vi "Clik.vi"(0 "refnum in":refnum<k7>, 1 "string in":string, 3 "错误输入":errorcluster) -> (7 "refnum out":refnum<k7>, 10 "错误输出":errorcluster)   [LabVIEW 2013]
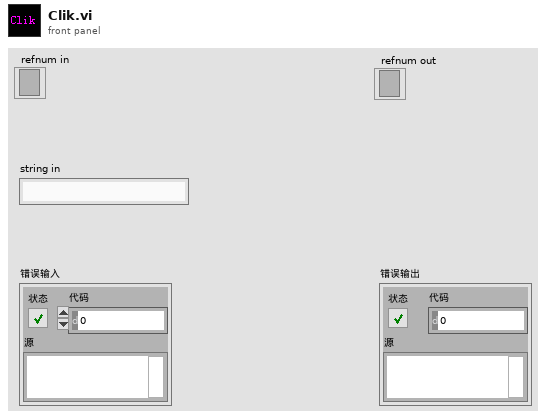
[diagram p1: front panel]
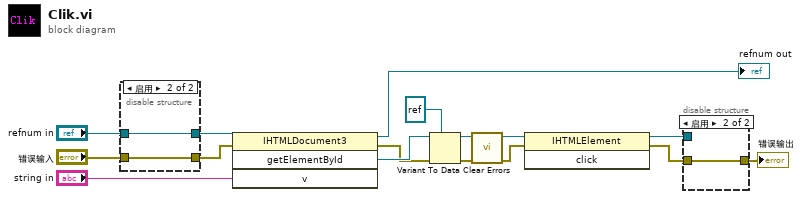
[diagram p0: block diagram]
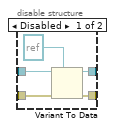
[diagram p2: hidden frame]
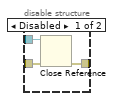
[diagram p3: hidden frame]
diagram:
  n1 = disable-structure shown="启用" {
    disable-tunnel: [w19 w22] -> w15
    disable-tunnel: "refnum in" -> [w18 w22]
    disable-tunnel: "错误输入" -> [w17 w21]
    disable-tunnel: [w16 w21] -> w6
    frame Disabled {
      n2 = Variant To Data(error in=w17, type=refnum<k7> refnum ("引用输出"), Variant=w18) -> (data=w19:refnum<k7>, error out=w16:errorcluster)
    }
    frame Enabled {
    }
  }
  n3 = invoke on="调用节点" class="IHTMLDocument3" method="getElementById"(reference=w15, error in=w6, "v"="string in") -> (reference out=→"refnum out":refnum<k7>, error out=w9:errorcluster, "getElementById"=w11:refnum<k7>)  [unwired: 1 in, 1 out]
  n4 = Variant To Data(error in=w9, type=refnum<k7> refnum ("引用输出"), Variant=w11) -> (data=w5:refnum<k7>, error out=w4:errorcluster)
  n5 = call <vilib>:"Clear Errors.vi"("error in (no error)"=w4) -> ("error out"=w1:errorcluster)  [unwired: 6 in]
  n6 = invoke on="调用节点" class="IHTMLElement" method="click"(reference=w5, error in=w1) -> (reference out=w3:refnum<k7>, error out=w2:errorcluster)  [unwired: 1 in, 1 out]
  n7 = disable-structure shown="启用" {
    disable-tunnel: [w25 w26] -> w8
    disable-tunnel: w3 -> [w24 _]
    disable-tunnel: w2 -> [w23 w26]
    frame Disabled {
      n8 = Close Reference(reference=w24, error in (no error)=w23) -> (error out=w25:errorcluster)
    }
    frame Enabled {
    }
  }
  "错误输出" <- w8
